vi "MGCC_StaEst_load_complex.vi"(1 "file path (dialog if empty)":path) -> (0 "Array 13":cdb[][](array[numeric]))   [LabVIEW 2016]
doc: "-----------------------------------------------------------------------------------------------------------------------\nCopyright <2019> <The University of Tennessee at Knoxville and the University of Tennessee Research Foundation>\nThis software is released under BSD-3 \nhttps://opensource.org/licenses/BSD-3-Clause \nAdditional license options available at https://utrf.tennessee.edu/industry/sample-agreements/\n-----------------------------------------------------------------------------------------------------------------------"
uses:
  <vilib>/Utility/file.llb/Read Delimited Spreadsheet (string).vi
panel:
  in  "Array 12":cdb[][](array[numeric])
  out "all rows":string[][](array[string])
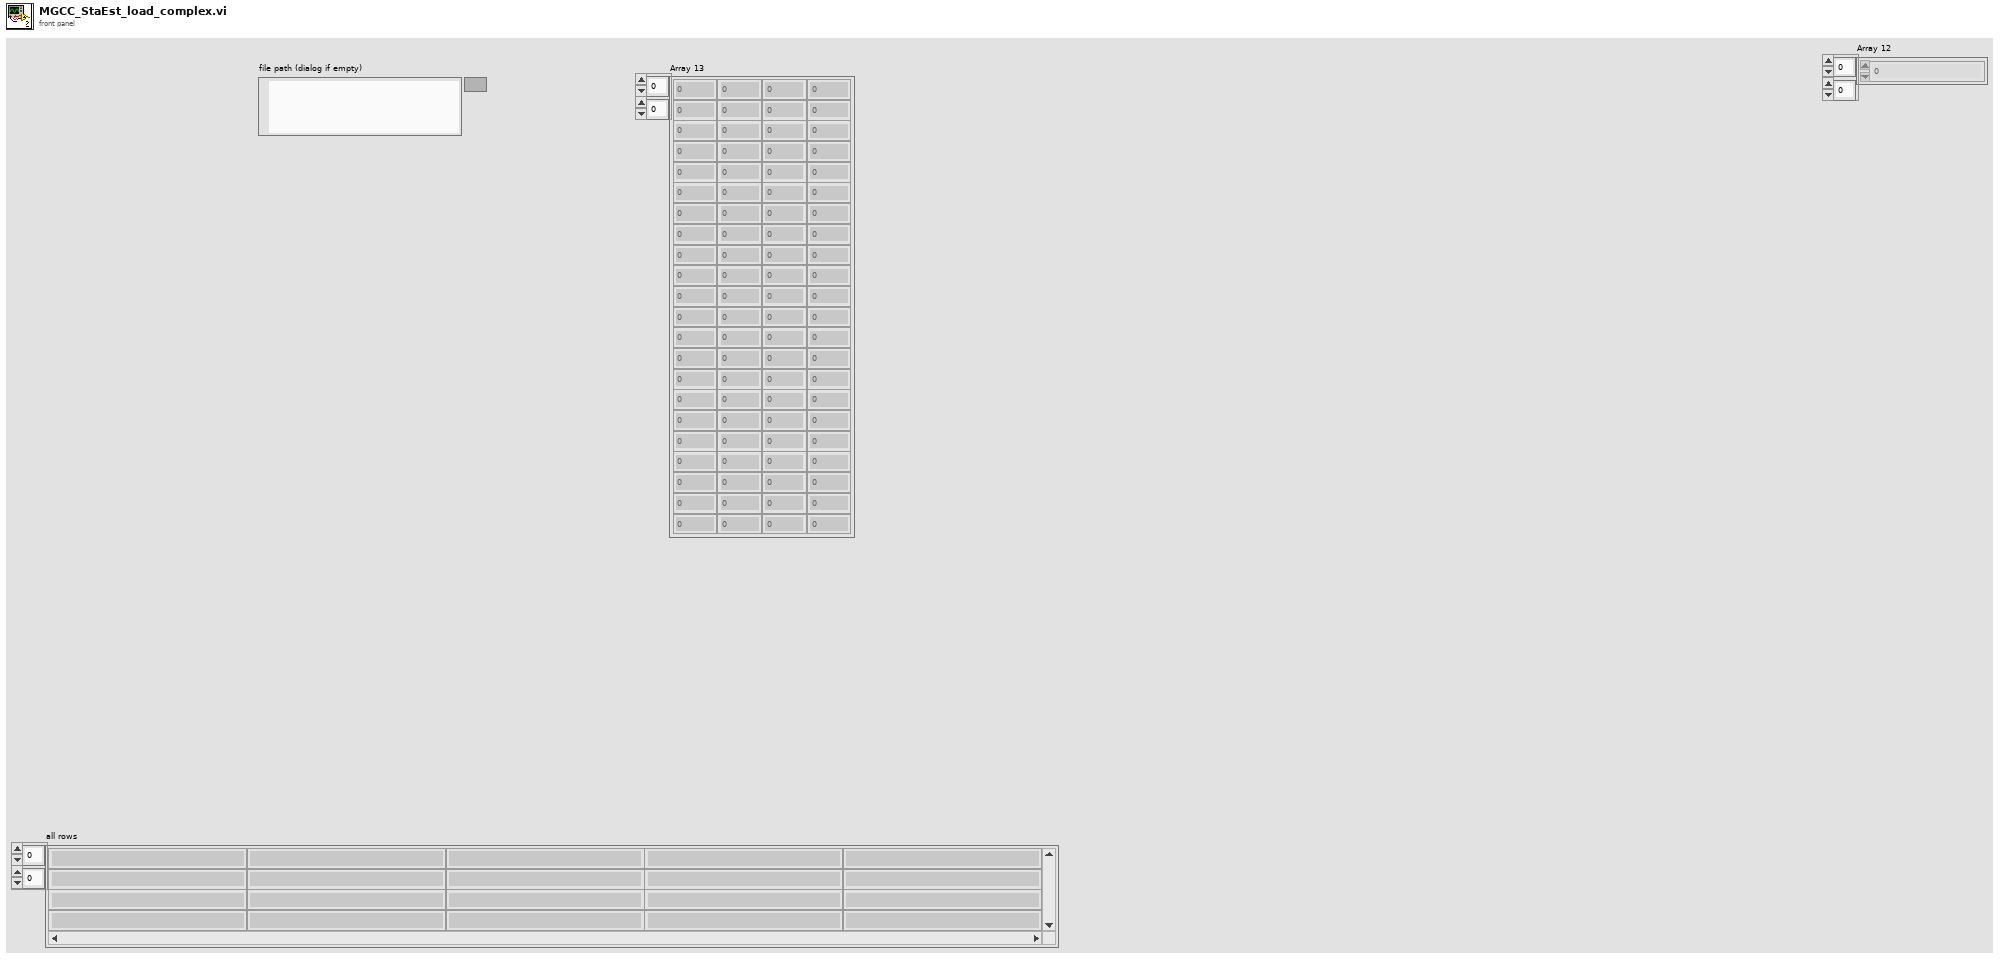
[diagram p1: front panel]
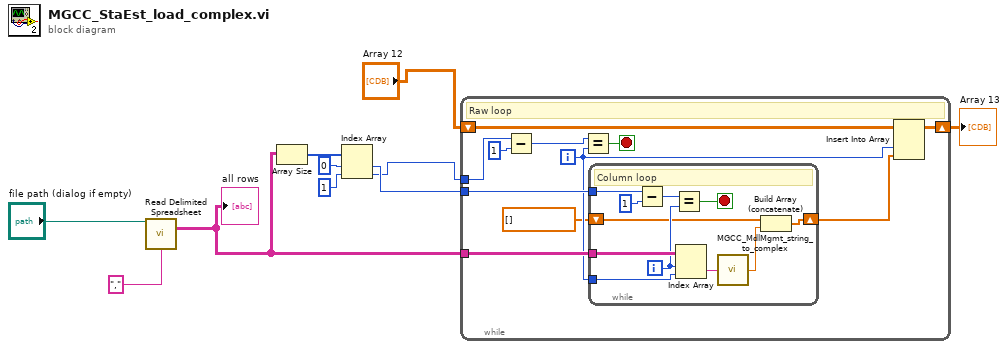
[diagram p0: block diagram]
diagram:
  n1 = call-poly <vilib>:"Read Delimited Spreadsheet.vi"("file path (dialog if empty)"="file path (dialog if empty)", "delimiter (\\t)"="," ("delimiter (\\t)")) -> ("all rows"=w6:string[][])  [unwired: 8 in, 5 out]
  "all rows" <- w6
  n2 = Array Size(array=w6) -> (size(s)=w10:i32[])
  n3 = Index Array(array=w10, index #1=0 ("index"), index #2=1 ("index")) -> (element #1=w8:i32, element #2=w4:i32)
  n4 = while {
    tunnel: w6 -> [w21]
    tunnel: w8 -> [w20]
    tunnel: w4 -> [w18]
    shift-right: [w14] -> w2
    shift-left: "Array 12" -> [w15]
    i -> [w13]
    stop <- w16 stop-if-true
    # "Raw loop"
    n5 = Subtract(x=w18, y=1) -> (x-y=w17:i32)
    n6 = Equal?(x=w17, y=w13) -> (x = y?=w16:bool)
    n7 = while {
      tunnel: w21 -> [w30]
      tunnel: w20 -> [w27]
      shift-right: [w22] -> w12
      shift-left: cdb[] [] -> [w28]
      tunnel: w13 -> [w23]
      i -> [w29]
      stop <- w32 stop-if-true
      # "Column loop"
      n8 = Subtract(x=w27, y=1) -> (x-y=w25:i32)
      n9 = Equal?(x=w25, y=w29) -> (x = y?=w32:bool)
      n10 = Index Array(array=w30, index (row)=w29, index (col)=w23) -> (element=w24:string)
      n11 = call "MGCC_MdlMgmt_string_to_complex.vi"("String Input"=w24) -> ("Complex Number"=w31:cdb)
      n12 = Build Array (concatenate)(w28, w31) -> (w22:cdb[])
    }
    n13 = Insert Into Array(array=w15, index (col)=w13, new element=w12) -> (w14:cdb[][])  [unwired: 1 in]
  }
  "Array 13" <- w2
